vi "unmarshalling.vi"(7 "Type":variant, 8 "error in (no error)":errorcluster, 10 "String":string, 11 "Serializer in":refnum<class "Serializer.LV-TOML.lvclass">) -> (0 "error out":errorcluster, 2 "Variant":variant, 3 "Serializer":refnum<class "Serializer.LV-TOML.lvclass">)   [LabVIEW 2020, in "OpenSerializer.LV-TOML.lvlib" / "Serializer.LV-TOML.lvclass"]
uses:
  Serializer.LV-TOML.lvclass
  <userlib>/LV-TOML/lib/LV-TOML.lvlib
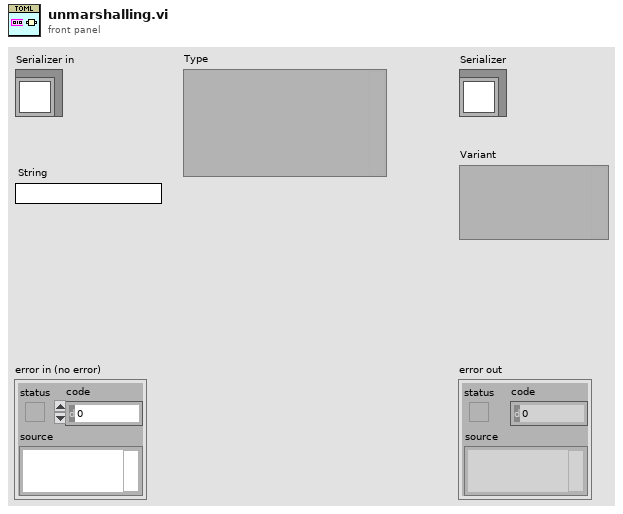
[diagram p1: front panel]
types:
  T1 = typedef "LV-TOML.lvlib/TOML Value.ctl" = cluster{"type":enum16{"Table", "Array", "String", "Integer", "Float", "Boolean", "Offset Date-Time", "Local Date-Time", "Local Date", "Local Time"}, "value":variant}
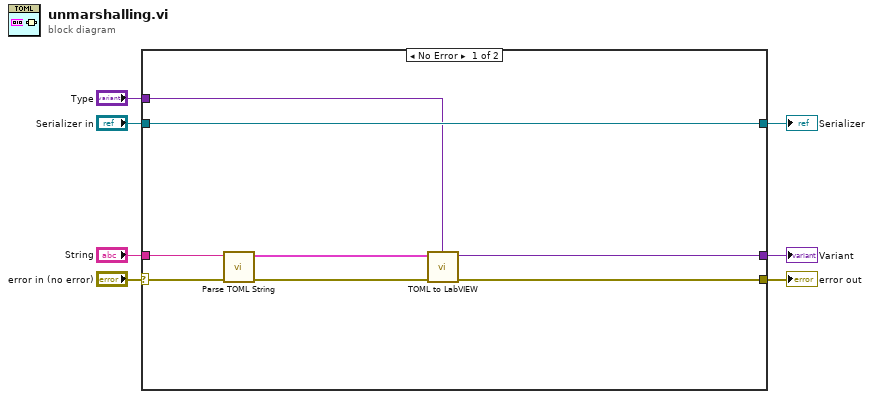
[diagram p0: block diagram]
diagram:
  n1 = case shown="No Error" "error in (no error)" {
    selector: "error in (no error)" -> [w14 w16]
    tunnel: "Serializer in" -> [w15 w17]
    tunnel: "String" -> [w13 _]
    tunnel: [w15 w17] -> w5
    tunnel: [w8 w16] -> w4
    tunnel: [w9 _] -> w3
    tunnel: "Type" -> [w10 _]
    frame No Error {
      n2 = call <userlib>:"Parse TOML String.vi"("error in (no error)"=w14, "String"=w13) -> ("error out"=w11:errorcluster, "Value"=w12:T1)  [unwired: 8 in]
      n3 = call <userlib>:"TOML to LabVIEW.vi"("Default Value"=w10, "error in (no error)"=w11, "TOML Value"=w12) -> ("error out"=w8:errorcluster, "LV Value"=w9:variant)  [unwired: 7 in]
    }
    frame Error {
    }
  }
  "error out" <- w4
  "Serializer" <- w5
  "Variant" <- w3
